vi "image_snap.vi"() -> ()   [LabVIEW 2020]
uses:
  <vilib>/userdefined/High Color/IMAQdx.ctl
  <vilib>/vision/driver/NI_Vision_Acquisition_Software.lvlib
panel:
  out "Image":T1(plugin-control)
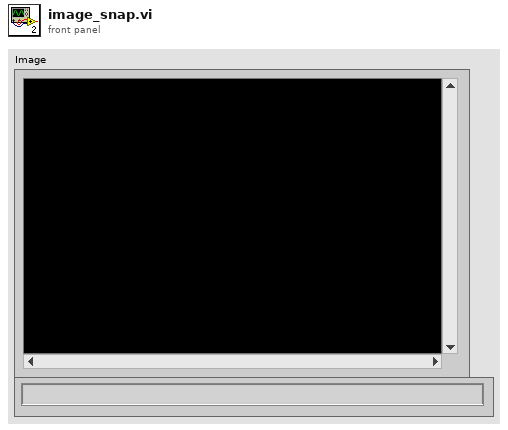
[diagram p1: front panel]
types:
  T1 = typedef "IMAQ Image.ctl" = refnum<image>
  T2 = typedef "IMAQdx.ctl" = refnum<k21>
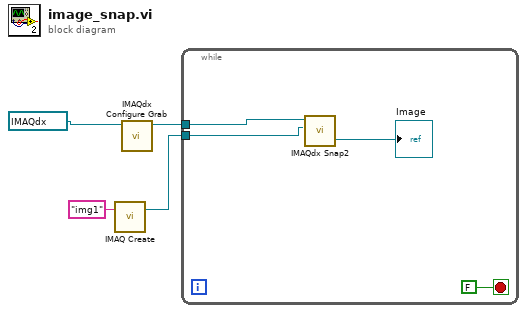
[diagram p0: block diagram]
diagram:
  n1 = call "IMAQ Create"("Image Name"="img1") -> ("New Image"=w1:T1)  [unwired: 4 in, 1 out]
  n2 = call <vilib>:"IMAQdx Configure Grab.vi"("Session In"=T2 "cam0") -> ("Session Out"=w2:T2)  [unwired: 9 in, 1 out]
  n3 = while {
    tunnel: w2 -> [w8]
    tunnel: w1 -> [w6]
    stop <- FALSE stop-if-true
    n4 = call <vilib>:"IMAQdx Snap2.vi"("Image In"=w6, "Session In"=w8) -> ("Image Out"=→"Image":T1)  [unwired: 7 in, 2 out]
  }
